vi "Configure Waveform Characteristics.vi"(0 "VISA resource name":refnum<visa-resource-name>, 1 "Period (0.001)":dbl=0.001, 2 "Frequency (1000 Hz)":dbl=1000.0, 3 "Noise (0 %)":dbl, 5 "Function Type (0: Sine)":i32(ring) items=["Sine", "Square", "Ramp", "Pulse", "Noise", "DC", "Sine Cardinal", "Exponential Rise", "Exponential Fall", "Cardiac", "Gaussian Pulse", "Arbitrary"], 7 "Setting Style (0: Frequency)":i32(ring) items=["Frequency", "Period"], 9 "Symmetry (50.0 %)":dbl=50.0, 11 "error in (no error)":errorcluster, 12 "Pulse Width (1E-6 S)":dbl=1e-06, 13 "Duty Cycle (50.0 %)":dbl=50.0, 14 "Waveform Generator Number (1: Waveform Generator 1)":i32(ring)=1 items=["Waveform Generator 1"=1, "Waveform Generator 2"=2]) -> (4 "VISA resource name out":refnum<visa-resource-name>, 15 "error out":errorcluster)   [LabVIEW 2016, in "Agilent 2000 3000 X-Series.lvlib"]
doc: "Configures the waveform paramter of waveform generator."
uses:
  Agilent 2000 3000 X-Series.lvlib
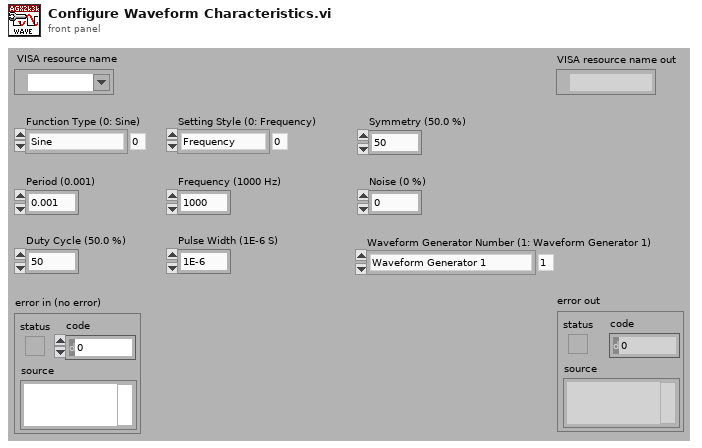
[diagram p1: front panel]
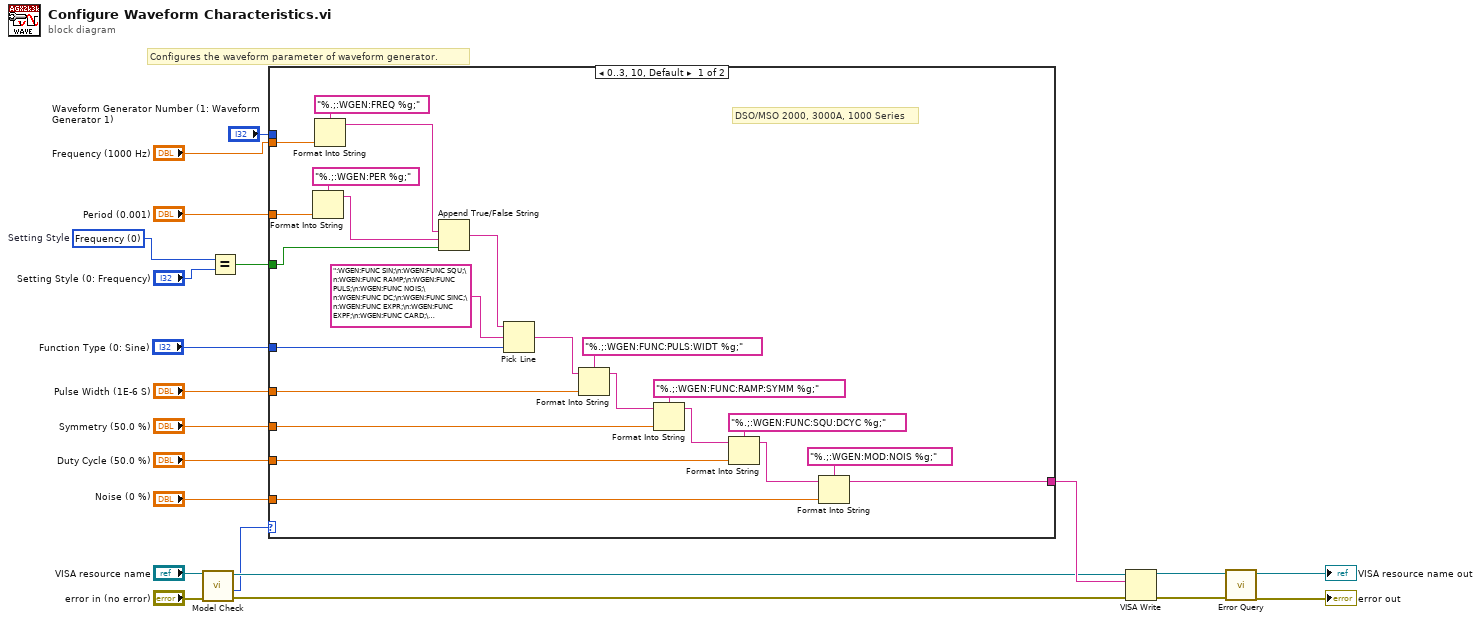
[diagram p0: block diagram]
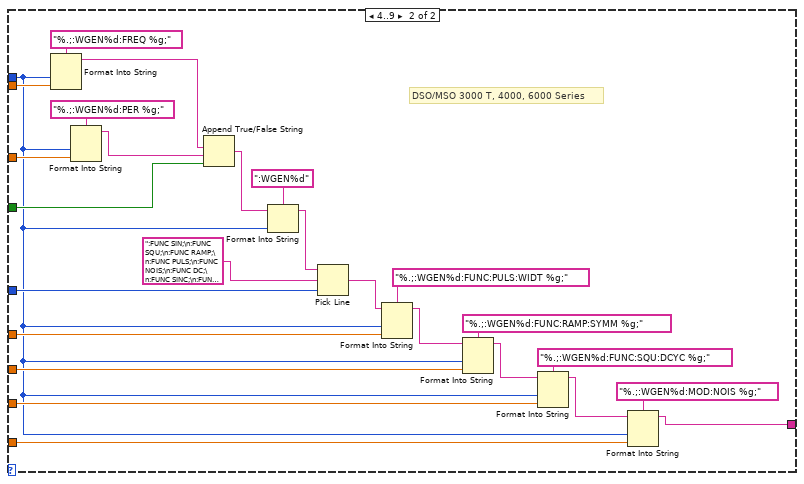
[diagram p2: hidden frame]
diagram:
  w10 = 0 items=["Frequency", "Period"]  # Setting Style
  # "Configures the waveform parameter of waveform generator."
  n1 = call "Model Check.vi"("error in (no error)"="error in (no error)", "VISA resource name"="VISA resource name") -> ("error out"=w3:errorcluster, "Model"=w1:i32, "VISA resource name out"=w4:refnum<visa-resource-name>)  [unwired: 7 out]
  n2 = Equal?(x=w10, y="Setting Style (0: Frequency)") -> (x = y?=w9:bool)
  n3 = case shown="0..3, 10, Default" w1 {
    tunnel: "Frequency (1000 Hz)" -> [w43 w57]
    tunnel: "Period (0.001)" -> [w41 w56]
    tunnel: "Function Type (0: Sine)" -> [w39 w51]
    tunnel: "Pulse Width (1E-6 S)" -> [w36 w50]
    tunnel: "Symmetry (50.0 %)" -> [w33 w49]
    tunnel: "Duty Cycle (50.0 %)" -> [w30 w48]
    tunnel: w9 -> [w28 w55]
    tunnel: "Noise (0 %)" -> [w25 w47]
    tunnel: [w23 w46] -> w7
    tunnel: "Waveform Generator Number (1: Waveform Generator 1)" -> [_ w45]
    frame 0..3, 10, Default {
      # "DSO/MSO 2000, 3000A, 1000 Series"
      n4 = Format Into String(format string="%.;:WGEN:PER %g;", w41) -> (resulting string=w27:string)  [unwired: 2 in, 1 out]
      n5 = Format Into String(format string="%.;:WGEN:FREQ %g;", w43) -> (resulting string=w26:string)  [unwired: 2 in, 1 out]
      n6 = Append True/False String(1:w28, 2:w27, 3:w26) -> (0:w29:string)  [unwired: 1 out]
      n7 = Pick Line(string ("")=w29, multi-line string=":WGEN:FUNC SIN;\n:WGEN:FUNC SQU;\n:WGEN:FUNC RAMP;\n:WGEN:FUNC PULS;\n:WGEN:FUNC NOIS;\n:WGEN:FUNC DC;\n:WGEN:FUNC SINC;\n:WGEN:FUNC EXPR;\n:WGEN:FUNC EXPF;\n:WGEN:FUNC CARD;\n:WGEN:FUNC GAUS;\n:WGEN:FUNC ARB;", line index=w39) -> (output string=w38:string)
      n8 = Format Into String(format string="%.;:WGEN:FUNC:PULS:WIDT %g;", initial string=w38, w36) -> (resulting string=w35:string)  [unwired: 1 in, 1 out]
      n9 = Format Into String(format string="%.;:WGEN:FUNC:RAMP:SYMM %g;", initial string=w35, w33) -> (resulting string=w32:string)  [unwired: 1 in, 1 out]
      n10 = Format Into String(format string="%.;:WGEN:FUNC:SQU:DCYC %g;", initial string=w32, w30) -> (resulting string=w24:string)  [unwired: 1 in, 1 out]
      n11 = Format Into String(format string="%.;:WGEN:MOD:NOIS %g;", initial string=w24, w25) -> (resulting string=w23:string)  [unwired: 1 in, 1 out]
    }
    frame 4..9 {
      # "DSO/MSO 3000 T, 4000, 6000 Series"
      n12 = Format Into String(format string="%.;:WGEN%d:FREQ %g;", w45, w57) -> (resulting string=w60:string)  [unwired: 2 in, 1 out]
      n13 = Format Into String(format string="%.;:WGEN%d:PER %g;", w45, w56) -> (resulting string=w61:string)  [unwired: 2 in, 1 out]
      n14 = Append True/False String(1:w55, 2:w61, 3:w60) -> (0:w53:string)  [unwired: 1 out]
      n15 = Format Into String(format string=":WGEN%d", initial string=w53, w45) -> (resulting string=w52:string)  [unwired: 1 in, 1 out]
      n16 = Pick Line(string ("")=w52, multi-line string=":FUNC SIN;\n:FUNC SQU;\n:FUNC RAMP;\n:FUNC PULS;\n:FUNC NOIS;\n:FUNC DC;\n:FUNC SINC;\n:FUNC EXPR;\n:FUNC EXPF;\n:FUNC CARD;\n:FUNC GAUS;\n:FUNC ARB;", line index=w51) -> (output string=w67:string)
      n17 = Format Into String(format string="%.;:WGEN%d:FUNC:PULS:WIDT %g;", initial string=w67, w45, w50) -> (resulting string=w65:string)  [unwired: 1 in, 1 out]
      n18 = Format Into String(format string="%.;:WGEN%d:FUNC:RAMP:SYMM %g;", initial string=w65, w45, w49) -> (resulting string=w63:string)  [unwired: 1 in, 1 out]
      n19 = Format Into String(format string="%.;:WGEN%d:FUNC:SQU:DCYC %g;", initial string=w63, w45, w48) -> (resulting string=w59:string)  [unwired: 1 in, 1 out]
      n20 = Format Into String(format string="%.;:WGEN%d:MOD:NOIS %g;", initial string=w59, w45, w47) -> (resulting string=w46:string)  [unwired: 1 in, 1 out]
    }
  }
  n21 = VISA Write(VISA resource name=w4, write buffer=w7, error in (no error)=w3) -> (VISA resource name out=w15:refnum<visa-resource-name>, error out=w14:errorcluster)  [unwired: 1 out]
  n22 = call "Error Query.vi"("error in (no error)"=w14, "VISA resource name"=w15) -> ("error out"=→"error out":errorcluster, "VISA resource name out"=→"VISA resource name out":refnum<visa-resource-name>)  [unwired: 8 out]
